vi "change type for single diagram.vi"(8 "error in (no error)":errorcluster, 9 "old type":T1, 10 "new type":T1, 11 "Diagram in":refnum<vi>) -> ()   [LabVIEW 2013]
uses:
  tag bus/trunk/tag/Data Type.ctl
  tag bus/trunk/tag/tag descriptor.lvclass
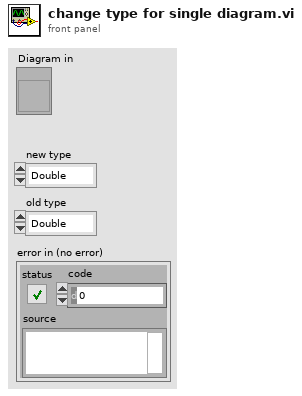
[diagram p1: front panel]
types:
  T1 = typedef "tag bus.lvlib/tag descriptor.lvclass/Data Type.ctl" = enum16{"Double", "Single", "I64", "I32", "I16", "I8", "U64", "U32", "U16", "U8", "Boolean", "String", "Array of Double", "Array of Single", "Array of I64", "Array of I32", "Array of I16", "Array of I8", "Array of U64", "Array of U32", "Array of U16", "Array of U8", "Array of Boolean", "Array of String"}
  T2 = cluster{"VIPath":path, "Menu Name":string, "Selector Name":string}[]
  T3 = cluster{"VIPath":path, "Menu Name":string, "Selector Name":string}
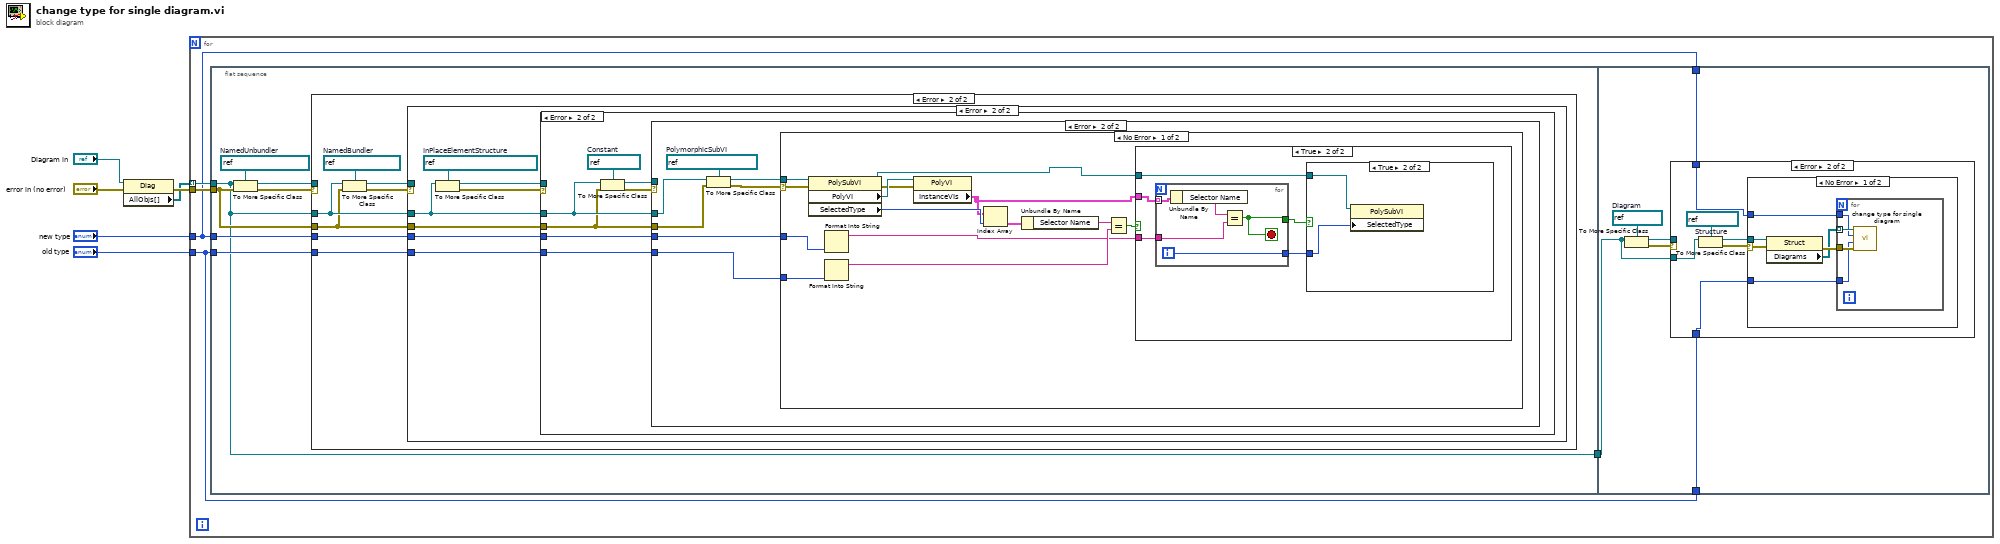
[diagram p0: block diagram]
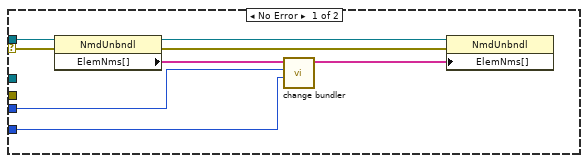
[diagram p2: hidden frame]
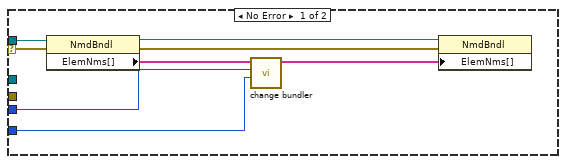
[diagram p3: hidden frame]
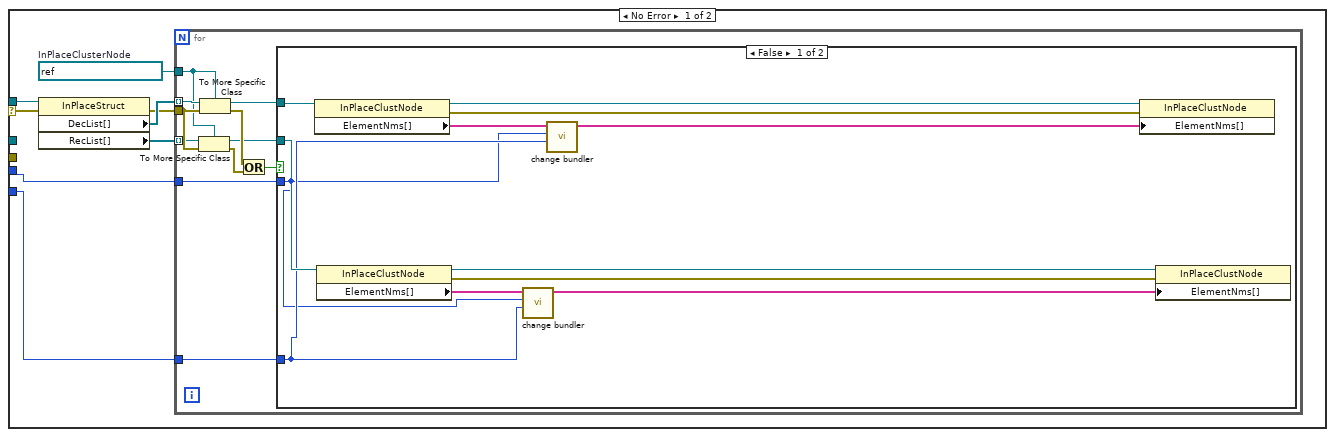
[diagram p4: hidden frame]
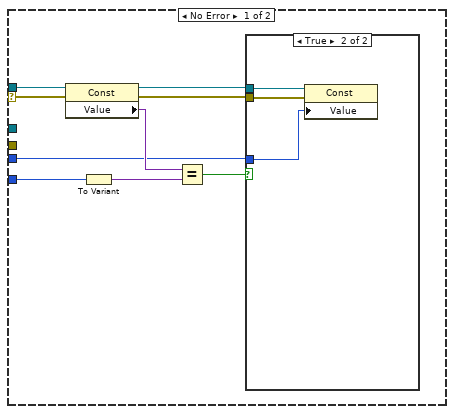
[diagram p6: hidden frame]
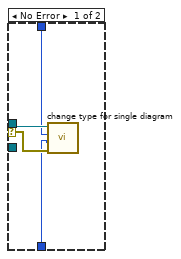
[diagram p11: hidden frame]
diagram:
  n1 = property class="Diag"(reference="Diagram in", error in="error in (no error)") -> (error out=w3:errorcluster, "AllObjs[]"=w2:refnum<vi>[])  [unwired: 1 out]
  n2 = for {
    tunnel: w2 -> [w11] mode=indexing
    tunnel: w3 -> [w10]
    tunnel: "old type" -> [w7]
    tunnel: "new type" -> [w8]
    n3 = flat-sequence {
      tunnel: w11 -> [w12]
      tunnel: w10 -> [w15]
      tunnel: w7 -> [w14]
      tunnel: w8 -> [w13]
      tunnel: [w12] -> w9
      tunnel: w9 -> [w132]
      tunnel: w8 -> [w134]
      tunnel: w7 -> [w133]
      frame #0 {
        w18 = refnum<vi> refnum  # NamedUnbundler
        n4 = To More Specific Class(target class=w18, reference=w12, error in=w15) -> (specific class reference=w16:refnum<vi>, error out=w17:errorcluster)
        n5 = case shown="Error" w17 {
          selector: w17 -> [w25 _]
          tunnel: w16 -> [w26 _]
          tunnel: w12 -> [_ w30]
          tunnel: w15 -> [_ w29]
          tunnel: w14 -> [w20 w28]
          tunnel: w13 -> [w19 w27]
          frame No Error {
            n6 = property class="NmdUnbndl"(reference=w26, error in=w25) -> (reference out=w24:refnum<vi>, error out=w23:errorcluster, "ElemNms[]"=w22:string[])
            n7 = call "change bundler.vi"("old data type"=w20, "new data type"=w19, "ElemNms[]"=w22) -> ("elemnames out"=w21:string[])  [unwired: 8 in]
            n8 = property class="NmdUnbndl"(reference=w24, error in=w23, "ElemNms[]"=w21) -> ()  [unwired: 2 out]
          }
          frame Error {
            w33 = refnum<vi> refnum  # NamedBundler
            n9 = To More Specific Class(target class=w33, reference=w30, error in=w29) -> (specific class reference=w31:refnum<vi>, error out=w32:errorcluster)
            n10 = case shown="Error" w32 {
              selector: w32 -> [w36 _]
              tunnel: w31 -> [w37 _]
              tunnel: w30 -> [_ w42]
              tunnel: w29 -> [_ w45]
              tunnel: w28 -> [w34 w44]
              tunnel: w27 -> [w35 w43]
              frame No Error {
                n11 = property class="NmdBndl"(reference=w37, error in=w36) -> (reference out=w40:refnum<vi>, error out=w39:errorcluster, "ElemNms[]"=w41:string[])
                n12 = call "change bundler.vi"("old data type"=w34, "new data type"=w35, "ElemNms[]"=w41) -> ("elemnames out"=w38:string[])  [unwired: 8 in]
                n13 = property class="NmdBndl"(reference=w40, error in=w39, "ElemNms[]"=w38) -> ()  [unwired: 2 out]
              }
              frame Error {
                w48 = refnum<vi> refnum  # InPlaceElementStructure
                n14 = To More Specific Class(target class=w48, reference=w42) -> (specific class reference=w46:refnum<vi>, error out=w47:errorcluster)  [unwired: 1 in]
                n15 = case shown="Error" w47 {
                  selector: w47 -> [w55 _]
                  tunnel: w46 -> [w56 _]
                  tunnel: w42 -> [_ w81]
                  tunnel: w45 -> [_ w80]
                  tunnel: w44 -> [w49 w83]
                  tunnel: w43 -> [w50 w82]
                  frame No Error {
                    w52 = refnum<vi> refnum  # InPlaceClusterNode
                    n16 = property class="InPlaceStruct"(reference=w56, error in=w55) -> (error out=w53:errorcluster, "DecList[]"=w54:refnum<vi>[], "RecList[]"=w51:refnum<vi>[])  [unwired: 1 out]
                    n17 = for {
                      tunnel: w54 -> [w67] mode=indexing
                      tunnel: w53 -> [w66]
                      tunnel: w52 -> [w64]
                      tunnel: w51 -> [w65] mode=indexing
                      tunnel: w50 -> [w58]
                      tunnel: w49 -> [w57]
                      n18 = To More Specific Class(target class=w64, reference=w65, error in=w66) -> (specific class reference=w59:refnum<vi>, error out=w62:errorcluster)
                      n19 = To More Specific Class(target class=w64, reference=w67, error in=w66) -> (specific class reference=w60:refnum<vi>, error out=w63:errorcluster)
                      n20 = Or(x=w63, y=w62) -> (x .or. y?=w61:bool)
                      n21 = case shown="False" w61 {
                        tunnel: w60 -> [w74 _]
                        tunnel: w59 -> [w75 _]
                        tunnel: w58 -> [w68 _]
                        tunnel: w57 -> [w69 _]
                        frame False {
                          n22 = property class="InPlaceClustNode"(reference=w74) -> (reference out=w79:refnum<vi>, error out=w78:errorcluster, "ElementNms[]"=w71:string[])  [unwired: 1 in]
                          n23 = property class="InPlaceClustNode"(reference=w75) -> (reference out=w76:refnum<vi>, error out=w77:errorcluster, "ElementNms[]"=w73:string[])  [unwired: 1 in]
                          n24 = call "change bundler.vi"("old data type"=w69, "new data type"=w68, "ElemNms[]"=w73) -> ("elemnames out"=w72:string[])  [unwired: 8 in]
                          n25 = call "change bundler.vi"("old data type"=w69, "new data type"=w68, "ElemNms[]"=w71) -> ("elemnames out"=w70:string[])  [unwired: 8 in]
                          n26 = property class="InPlaceClustNode"(reference=w79, error in=w78, "ElementNms[]"=w70) -> ()  [unwired: 2 out]
                          n27 = property class="InPlaceClustNode"(reference=w76, error in=w77, "ElementNms[]"=w72) -> ()  [unwired: 2 out]
                        }
                        frame True {
                          # "shouldnt ever happen if I understand ipestructs"
                        }
                      }
                    }
                  }
                  frame Error {
                    w86 = refnum<vi> refnum  # Constant
                    n28 = To More Specific Class(target class=w86, reference=w81, error in=w80) -> (specific class reference=w84:refnum<vi>, error out=w85:errorcluster)
                    n29 = case shown="Error" w85 {
                      selector: w85 -> [w94 _]
                      tunnel: w84 -> [w95 _]
                      tunnel: w83 -> [w93 w99]
                      tunnel: w82 -> [w87 w100]
                      tunnel: w81 -> [_ w103]
                      tunnel: w80 -> [_ w104]
                      frame No Error {
                        n30 = property class="Const"(reference=w95, error in=w94) -> (reference out=w89:refnum<vi>, error out=w88:errorcluster, "Value"=w92:variant)
                        n31 = To Variant(anything=w93) -> (Variant=w91:variant)
                        n32 = Equal?(x=w92, y=w91) -> (x = y?=w90:bool)
                        n33 = case shown="True" w90 {
                          tunnel: w89 -> [_ w98]
                          tunnel: w88 -> [_ w97]
                          tunnel: w87 -> [_ w96]
                          frame False {
                          }
                          frame True {
                            n34 = property class="Const"(reference=w98, error in=w97, "Value"=w96) -> ()  [unwired: 2 out]
                          }
                        }
                      }
                      frame Error {
                        w105 = refnum<vi> refnum  # PolymorphicSubVI
                        n35 = To More Specific Class(target class=w105, reference=w103, error in=w104) -> (specific class reference=w102:refnum<vi>, error out=w101:errorcluster)
                        n36 = case shown="No Error" w101 {
                          selector: w101 -> [w118 _]
                          tunnel: w102 -> [w119 _]
                          tunnel: w100 -> [w113 _]
                          tunnel: w99 -> [w112 _]
                          frame No Error {
                            n37 = property class="PolySubVI"(reference=w119, error in=w118) -> (reference out=w108:refnum<vi>, error out=w116:errorcluster, "PolyVI"=w117:refnum<vi>, "SelectedType"=w107:i32)
                            n38 = Format Into String(w113) -> (resulting string=w109:string)  [unwired: 3 in, 1 out]
                            n39 = Format Into String(w112) -> (resulting string=w111:string)  [unwired: 3 in, 1 out]
                            n40 = property class="PolyVI"(reference=w117, error in=w116) -> ("InstanceVIs"=w106:T2)  [unwired: 2 out]
                            n41 = Index Array(array=w106, index=w107) -> (element=w115:T3)
                            n42 = Unbundle By Name(w115) -> ("Selector Name"=w114:string)
                            n43 = Equal?(x=w114, y=w111) -> (x = y?=w110:bool)
                            n44 = case shown="True" w110 {
                              tunnel: w106 -> [_ w124]
                              tunnel: w109 -> [_ w123]
                              tunnel: w108 -> [_ w121]
                              frame False {
                              }
                              frame True {
                                n45 = for {
                                tunnel: w124 -> [w131] mode=indexing
                                tunnel: w123 -> [w129]
                                tunnel: [w128] -> w122
                                tunnel: [w127] -> w120
                                i -> [w127]
                                stop <- w128 stop-if-true
                                n46 = Unbundle By Name(w131) -> ("Selector Name"=w130:string)
                                n47 = Equal?(x=w130, y=w129) -> (x = y?=w128:bool)
                                }
                                n48 = case shown="True" w122 {
                                tunnel: w121 -> [_ w126]
                                tunnel: w120 -> [_ w125]
                                frame False {
                                }
                                frame True {
                                n49 = property class="PolySubVI"(reference=w126, "SelectedType"=w125) -> ()  [unwired: 1 in, 2 out]
                                }
                                }
                              }
                            }
                          }
                          frame Error {
                          }
                        }
                      }
                    }
                  }
                }
              }
            }
          }
        }
      }
      frame #1 {
        w137 = refnum<vi> refnum  # Diagram
        n50 = To More Specific Class(target class=w137, reference=w132) -> (specific class reference=w135:refnum<vi>, error out=w136:errorcluster)  [unwired: 1 in]
        n51 = case shown="Error" w136 {
          selector: w136 -> [w140 _]
          tunnel: w135 -> [w141 _]
          tunnel: w134 -> [w139 w143]
          tunnel: w133 -> [w138 w142]
          tunnel: w132 -> [_ w146]
          frame No Error {
            n52 = call "change type for single diagram.vi"("error in (no error)"=w140, "old type"=w138, "new type"=w139, "Diagram in"=w141) -> ()  [unwired: 8 in]
          }
          frame Error {
            w147 = refnum<vi> refnum  # Structure
            n53 = To More Specific Class(target class=w147, reference=w146) -> (specific class reference=w144:refnum<vi>, error out=w145:errorcluster)  [unwired: 1 in]
            n54 = case shown="No Error" w145 {
              selector: w145 -> [w152 _]
              tunnel: w144 -> [w153 _]
              tunnel: w143 -> [w149 _]
              tunnel: w142 -> [w148 _]
              frame No Error {
                n55 = property class="Struct"(reference=w153, error in=w152) -> (error out=w151:errorcluster, "Diagrams"=w150:refnum<vi>[])  [unwired: 1 out]
                n56 = for {
                  tunnel: w151 -> [w157]
                  tunnel: w150 -> [w156] mode=indexing
                  tunnel: w149 -> [w155]
                  tunnel: w148 -> [w154]
                  n57 = call "change type for single diagram.vi"("error in (no error)"=w157, "old type"=w154, "new type"=w155, "Diagram in"=w156) -> ()  [unwired: 8 in]
                }
              }
              frame Error {
              }
            }
          }
        }
      }
    }
  }
